vi "Initalize OPC UA.vi"(8 "error in (no error)":errorcluster, 11 "SM EOL Station Actor in":refnum<class "OPC Server.lvclass">) -> (0 "error out":errorcluster, 3 "SM EOL Station Actor out":refnum<class "OPC Server.lvclass">)   [LabVIEW 2021, in "OPC Server.lvlib" / "OPC Server.lvclass"]
uses:
  OPC Server.lvclass
  <vilib>/OPCUA/controls/Supported Security Policies.ctl
  OPC Server.lvclass/OPC Server.ctl
  <vilib>/OPCUA/NI OPC UA Server.lvlib
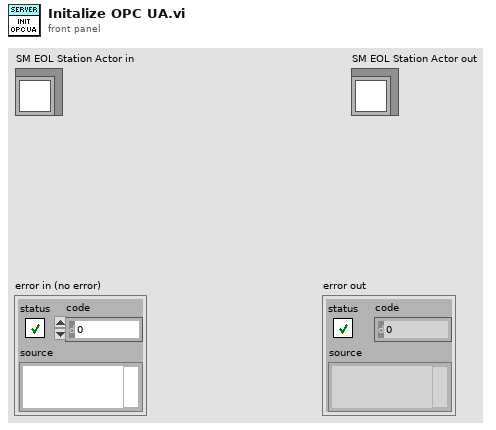
[diagram p1: front panel]
types:
  T1 = typedef "Supported Security Policies.ctl" = cluster{"None":bool, "Sign with Basic128Rsa15":bool, "Sign and Encrypt with Basic128Rsa15":bool, "Sign with Basic256":bool, "Sign and Encrypt with Basic256":bool}
  T2 = typedef "OPC UA Server Refnum.ctl" = refnum<k21>
  T3 = typedef "NodeId.ctl" = string
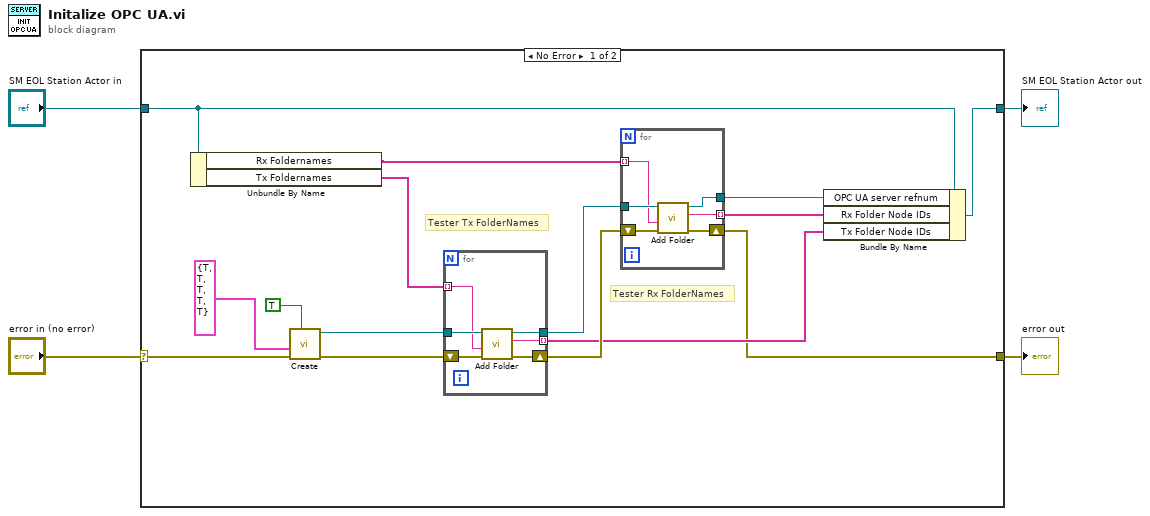
[diagram p0: block diagram]
diagram:
  n1 = case shown="No Error" "error in (no error)" {
    selector: "error in (no error)" -> [w19 w33]
    tunnel: [w6 w33] -> w3
    tunnel: [w18 w32] -> w1
    tunnel: "SM EOL Station Actor in" -> [w17 w32]
    frame No Error {
      # "Tester Rx FolderNames"
      # "Tester Tx FolderNames"
      n2 = Unbundle By Name(w17) -> ("Rx Foldernames"=w13:string[], "Tx Foldernames"=w14:string[])
      n3 = call <vilib>:"Create.vi"("trust all clients (F)"=TRUE, "error in (no error)"=w19, "supported security policies (None)"=T1 {"None"=TRUE, "Sign with Basic128Rsa15"=TRUE, "Sign and Encrypt with Basic128Rsa15"=TRUE, "Sign with Basic256"=TRUE, "Sign and Encrypt with Basic256"=TRUE}) -> ("error out"=w12:errorcluster, "OPC UA server refnum out"=w10:T2)  [unwired: 6 in, 1 out]
      n4 = for {
        tunnel: [w29] -> w7 mode=indexing
        tunnel: w14 -> [w28] mode=indexing
        shift-right: [w27] -> w11
        shift-left: w12 -> [w31]
        tunnel: w10 -> [w30]
        tunnel: [w26] -> w9
        n5 = call <vilib>:"Add Folder.vi"("error in (no error)"=w31, "folder name"=w28, "OPC UA server refnum in"=w30) -> ("error out"=w27:errorcluster, "folder node ID"=w29:T3, "OPC UA server refnum out"=w26:T2)  [unwired: 5 in]
      }
      n6 = for {
        tunnel: [w22] -> w8 mode=indexing
        tunnel: w13 -> [w21] mode=indexing
        shift-right: [w20] -> w6
        shift-left: w11 -> [w25]
        tunnel: w9 -> [w24]
        tunnel: [w23] -> w5
        n7 = call <vilib>:"Add Folder.vi"("error in (no error)"=w25, "folder name"=w21, "OPC UA server refnum in"=w24) -> ("error out"=w20:errorcluster, "folder node ID"=w22:T3, "OPC UA server refnum out"=w23:T2)  [unwired: 5 in]
      }
      n8 = Bundle By Name(cluster=w17, "OPC UA server refnum"=w5, "Rx Folder Node IDs"=w8, "Tx Folder Node IDs"=w7) -> (w18:refnum<class "OPC Server.lvclass">)
    }
    frame Error {
    }
  }
  "error out" <- w3
  "SM EOL Station Actor out" <- w1
